vi "Productos.vi"(8 "error in (no error)":errorcluster, 10 "Producto":dbl, 11 "Mensajes in":refnum<class "Mensajes.lvclass">) -> (0 "error out":errorcluster, 3 "Mensajes out":refnum<class "Mensajes.lvclass">)   [LabVIEW 2020, in "Mensajes.lvlib" / "Mensajes.lvclass"]
uses:
  Mensajes.lvclass
  Mensajes.lvclass/Mensajes.ctl
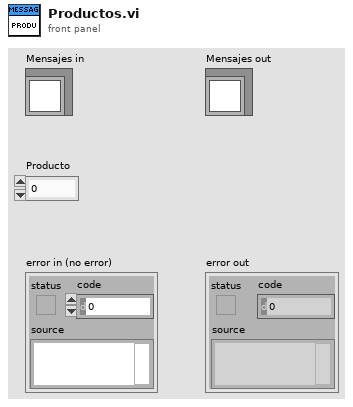
[diagram p1: front panel]
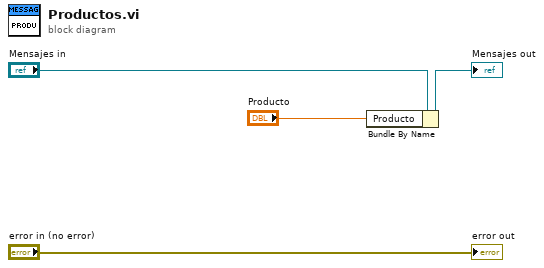
[diagram p0: block diagram]
diagram:
  n1 = Bundle By Name(cluster="Mensajes in", "Producto"="Producto") -> (→"Mensajes out":refnum<class "Mensajes.lvclass">)
  "error out" <- "error in (no error)"
